vi "ULx Cont Gen Voltage Wfm-Int Clk.vi"() -> ()   [LabVIEW 2015]
doc: "I. Description:\nThis example demonstrates how to output a continuous periodic waveform using an internal sample clock.\n\nII. Instructions for Running:\n1. Select the Physical Channel to correspond to where your signal is output on the DAQ device.\n2. Enter the Minimum and Maximum Voltage Ranges\n3. Specify the Desired Frequency of the output Waveform\n4. Enter the Waveform Information. See the documentation of the Waveform Buffer Generation SubVI for information on each parameter.\n\nIII. Block Diagram Steps:\n1. Create an Analog Output Voltage channel.\n2. Call the DAQmx Timing (Use Waveform) VI which sets the sample clock rate based on the input waveform parameters, and set the sample mode to Continuous.\n3. Write the waveform to the output buffer.\n4. Call the Start VI.\n5. Loop continuously until the user presses the Stop button. Check for errors every 100 ms using the Is Task Done? VI\n6. Clear the Task\n7. Use the popup dialog box to display an error or warning if any.\n\nIV. I/O Connections Overview:\nMake sure your signal output terminal matches the Physical Channel I/O Control. For further connection information, refer to your hardware reference manual."
uses:
  <vilib>/Utility/error.llb/DialogType.ctl
  <vilib>/ULx/Create Channel.llb/ULx Create Channel (AO-Voltage-Basic).vi
  <vilib>/ULx/Timing.llb/ULx Timing (Use Waveform).vi
  <vilib>/ULx/Write.llb/ULx Write (Analog Wfm 1Chan NSamp).vi
panel:
  in  "Wirite Timeout":dbl=10.0 format="%0.2f"
  in  "Max. Sample Clock Rate":dbl=1000.0 caption="Desired Sample Clock Rate" format="%.2f"
  out "error out":errorcluster
  out "Sample Clock Rate":dbl caption="Desired Sample Clock Rate" format="%.2f"
  in  "Offset":dbl format="%0.2p"
  in  "physical channel":refnum<k21>="Dev0/Ao0"
  in  "Cycles per Buffer":i32=10
  in  "Waveform Type":T1(ring)
  in  "Desired Frequency":dbl=10.0 format="%.2f"
  in  "Samples per Buffer":dbl=6400.0
  in  "Amplitude":dbl=1.0 format="%0.2p"
  out "Waveform Graph":waveform(dbl)(graph)={"t0"=timestamp(0 s since 1904-01-01), "dt"=0.001, "Y"=[]} caption="Output Waveform"
  in  "Minimum Value":dbl=-10.0 format="%0.2f"
  in  "Maximum Value":dbl=10.0 format="%0.2f"
  in  "stop":bool
  # "For instructions, select Help>>Show Context Help"
  # "Channel Parameters"
  # "Timing Parameters"
  # "Waveform Information"
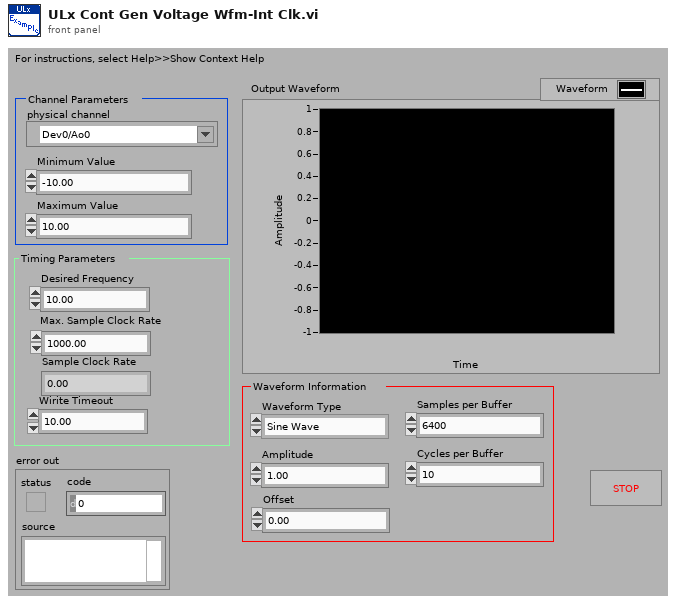
[diagram p1: front panel]
types:
  T1 = enum16{"Sine Wave", "Triangle Wave", "Square Wave", "Sawtooth Wave"}
  T2 = typedef "DialogType.ctl" = u16
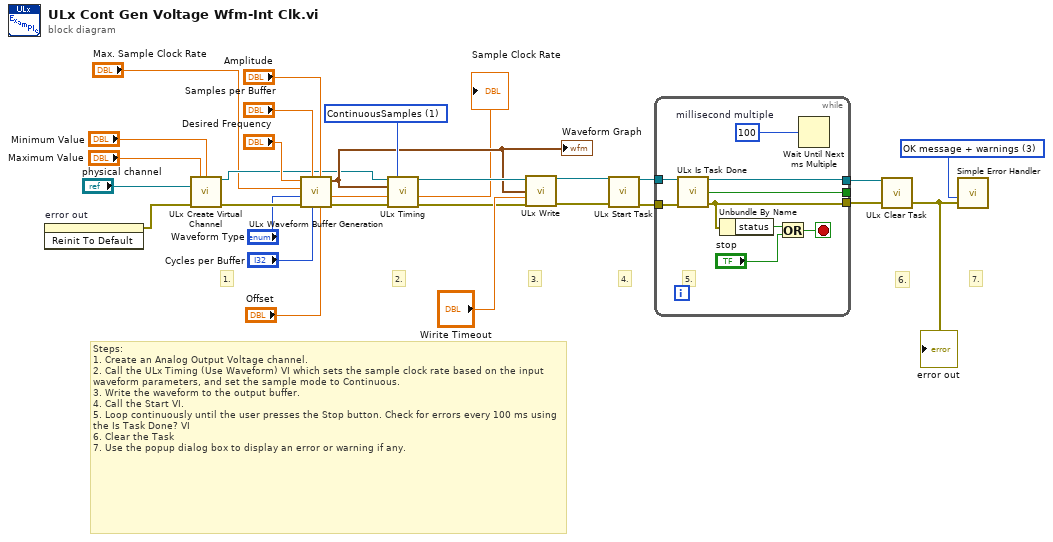
[diagram p0: block diagram]
diagram:
  w8 = 1 items=["FiniteSamples", "ContinuousSamples"] ("sample mode")
  w18 = T2 3 items=["no dialog", "OK message", "continue or stop message", "OK message + warnings", "continue/stop + warnings"] ("type of dialog (OK msg:1)")
  # "7."
  # "6."
  # "Steps: \n1. Create an Analog Output Voltage channel.\n2. Call the ULx Timing (Use Waveform) VI which sets the sample clock rate based on the input waveform parameters, and set the sample mode to Continuous.\n3. Write the waveform to the output buffer.\n4. Call the Start VI.\n5. Loop continuously until the user presses the Stop button. Check for errors every 100 ms using the Is Task Done? VI\n6. Clear the Task\n7. Use the popup dialog box to display an error or warning if any."
  # "4."
  # "3."
  # "2."
  # "1."
  n1 = invoke on="error out" class="Clust (strict)" method="Reinit To Default"() -> (error out=w2:errorcluster)  [unwired: 3 in, 2 out]
  n2 = call-poly <vilib>:"ULx Create Virtual Channel.vi"("maximum value"="Maximum Value", "minimum value"="Minimum Value", "physical channels"="physical channel", "error in"=w2) -> ("task out"=w5:refnum<k24>, "error out"=w14:errorcluster)  [unwired: 10 in]
  n3 = call "ULx Waveform Buffer Generation.vi"("Offset"="Offset", "Amplitude"="Amplitude", "Cycles per Buffer"="Cycles per Buffer", "Samples per Buffer"="Samples per Buffer", "error in (no error)"=w14, "Waveform Type"="Waveform Type", "Max. Sample Clock Rate"="Max. Sample Clock Rate", "Frequency"="Desired Frequency") -> ("error out"=w15:errorcluster, "Sample Clock Rate"=→"Sample Clock Rate":dbl, "Waveform"=w6:waveform(dbl))  [unwired: 1 in]
  "Waveform Graph" <- w6
  n4 = call-poly <vilib>:"ULx Timing.vi"("task in"=w5, "sample mode"=w8, "waveform"=w6, "error in"=w15) -> ("task out"=w21:refnum<k24>, "error out"=w20:errorcluster)  [unwired: 10 in]
  n5 = call-poly <vilib>:"ULx Write.vi"("task in"=w21, "data"=w6, "timeout"="Wirite Timeout", "error in"=w20) -> ("task out"=w25:refnum<k24>, "error out"=w24:errorcluster)  [unwired: 9 in, 1 out]
  n6 = call <vilib>:"ULx Start Task.vi"("task in"=w25, "error in"=w24) -> ("task out"=w19:refnum<k24>, "error out"=w22:errorcluster)  [unwired: 12 in]
  n7 = while {
    tunnel: w19 -> [w37]
    tunnel: [w36] -> w17
    tunnel: w22 -> [w35]
    tunnel: [w34] -> w16
    tunnel: [w29] -> _
    stop <- w32 stop-if-true
    w33 = u32 100  # millisecond multiple
    # "5."
    n8 = call <vilib>:"ULx Is Task Done.vi"("task in"=w37, "error in"=w35) -> ("task out"=w36:refnum<k24>, "task done?"=w29:bool, "error out"=w34:errorcluster)  [unwired: 11 in]
    n9 = Unbundle By Name(w34) -> ("status"=w31:bool)
    n10 = Or(x=w31, y="stop") -> (x .or. y?=w32:bool)
    n11 = Wait Until Next ms Multiple(millisecond multiple=w33) -> ()  [unwired: 1 out]
  }
  n12 = call <vilib>:"ULx Clear Task.vi"("task in"=w17, "error in"=w16) -> ("error out"=w28:errorcluster)  [unwired: 13 in]
  "error out" <- w28
  n13 = call <vilib>:"Simple Error Handler.vi"("type of dialog (OK msg:1)"=w18, "error in (no error)"=w28) -> ()  [unwired: 3 in, 5 out]
